vi "DAQ_Vibration (SubVI).vi"(8 "error in (no error)":errorcluster, 11 "output cluster":T1) -> (0 "error out":errorcluster)   [LabVIEW 2016]
uses:
  Que Cluster TD.ctl
  Que Attributes TD.ctl
  Que enum td.ctl
  Vibration data TD.ctl
  <vilib>/DAQmx/read.llb/DAQmx Read (Analog 2D DBL NChan NSamp).vi
  <vilib>/DAQmx/miscellaneous.llb/DAQmx Fill In Error Info.vi
  <resource>/objmgr/daqmx.rc
panel:
  out "Vibration_2":dbl[][](graph)
  out "Vibration_1":dbl[][](graph)
  in  "samples per read operation":i32=2560
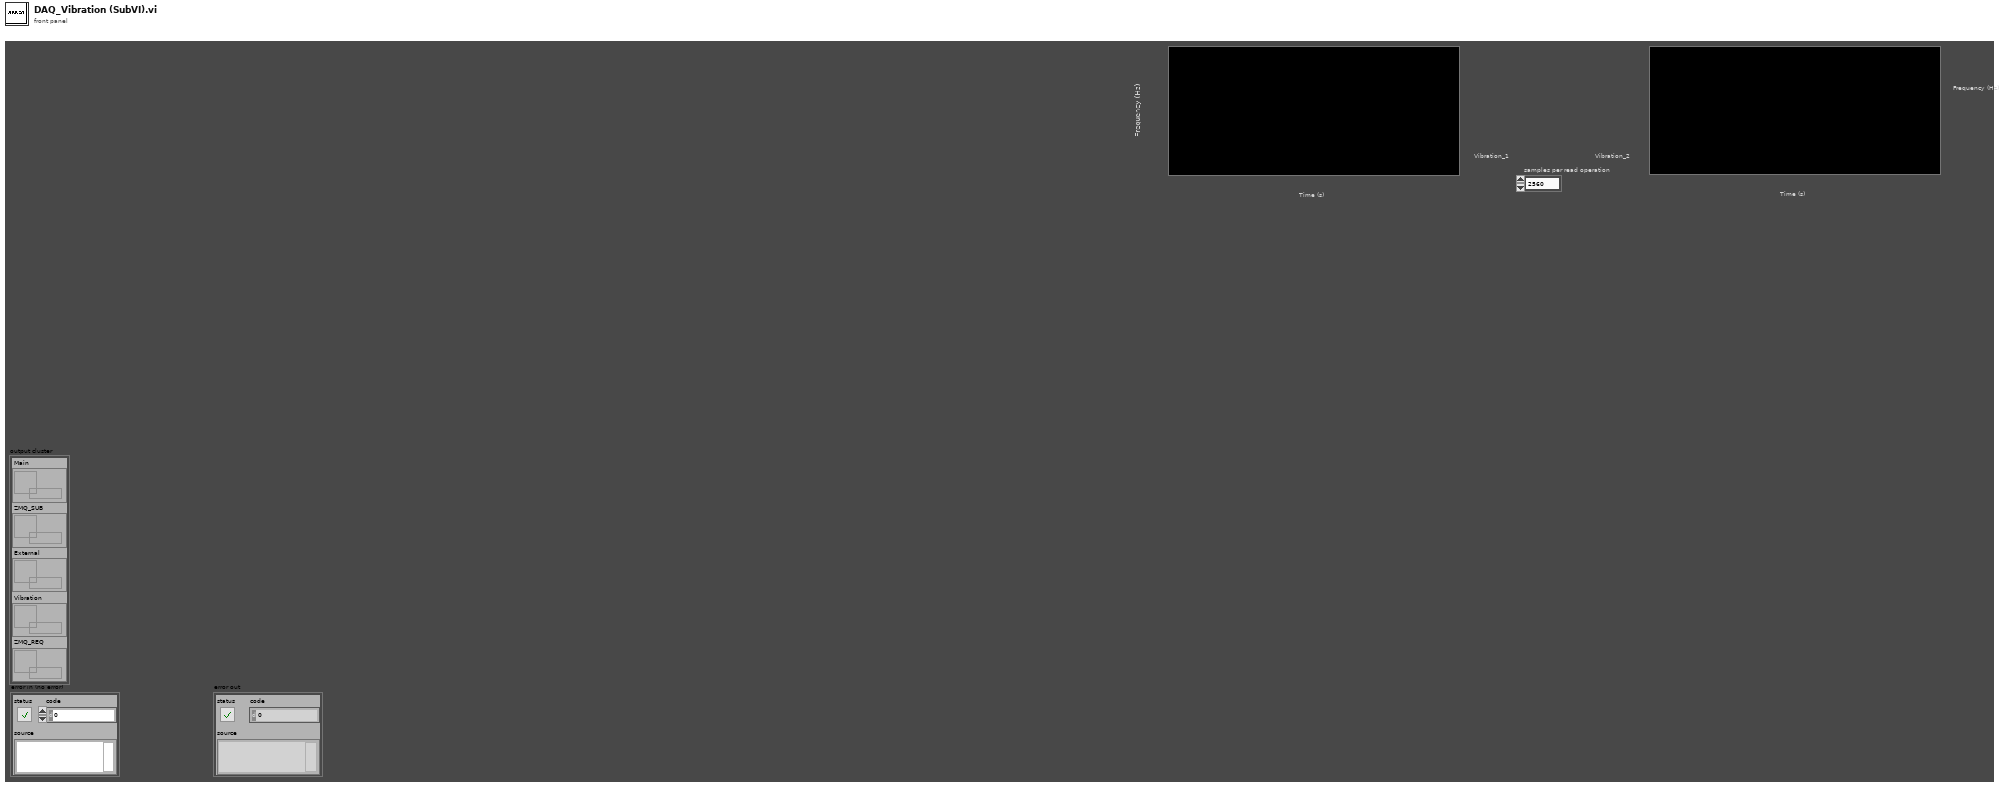
[diagram p1: front panel]
types:
  T1 = typedef "Que Cluster TD.ctl" = cluster{"Main":refnum<queue>, "ZMQ_SUB":refnum<queue>, "External":refnum<queue>, "Vibration":refnum<queue>, "ZMQ_REQ":refnum<queue>}
  T2 = typedef "Vibration data TD.ctl" = cluster{"# samples":i32, "Vibration_1":dbl[], "Vibration_2":dbl[], "Connected?":bool, "Logging?":bool, "TimeStamp":dbl, "Data":dbl[][], "LogFilePath":path}
  T3 = typedef "Que Attributes TD.ctl" = cluster{"Que States":T4, "String":string, "Boolean":bool, "Double":dbl, "U16":u16}
  T4 = typedef "Que enum td.ctl" = enum16{"Stop", "Start", "Update D_HW", "Initialize", "Exit", "Read", "Write", "Plot", "Log", "Stop Log", "Start Log", "Wait"}
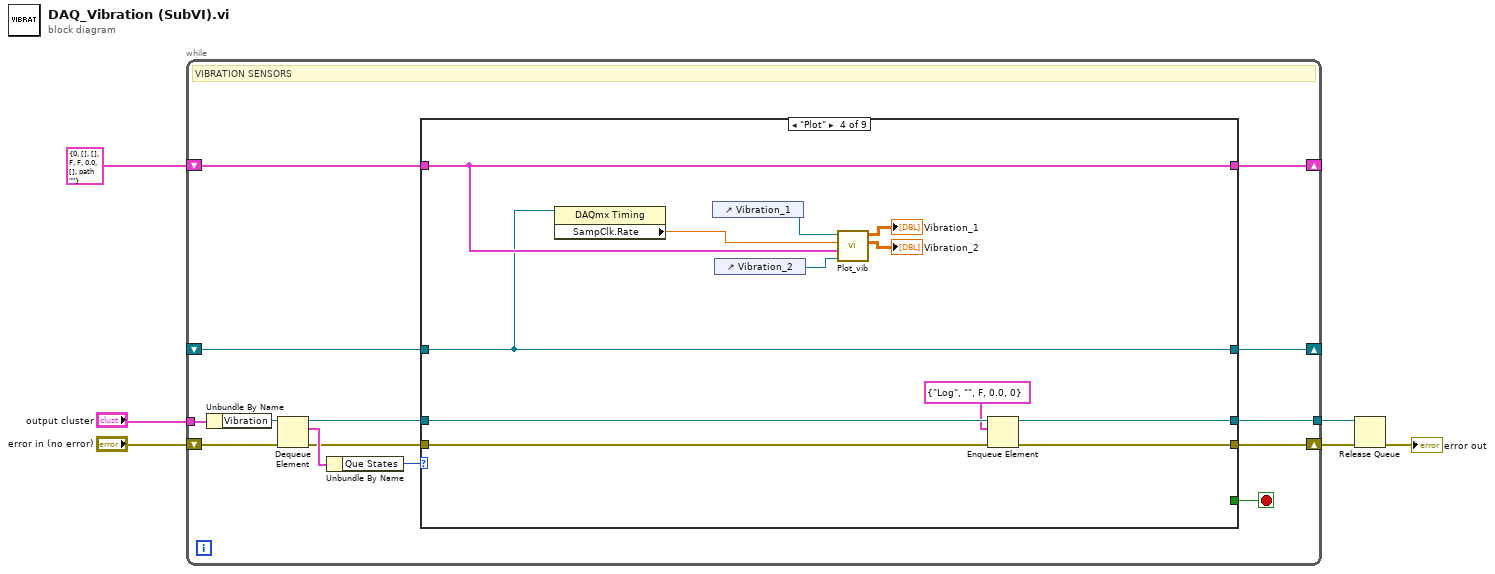
[diagram p0: block diagram]
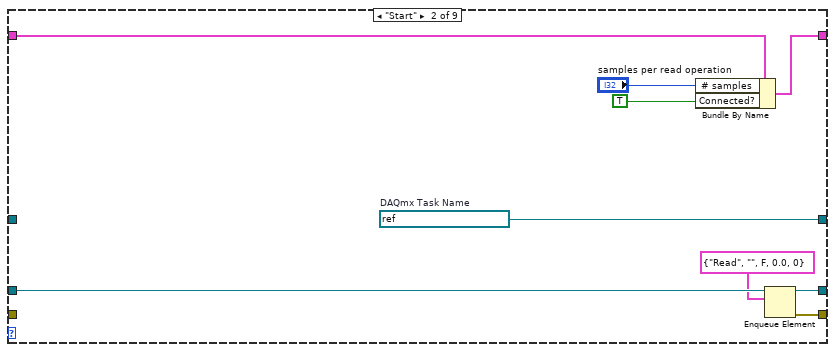
[diagram p3: hidden frame]
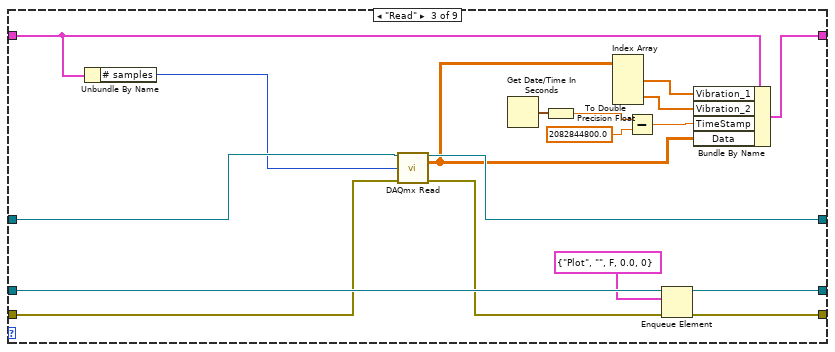
[diagram p4: hidden frame]
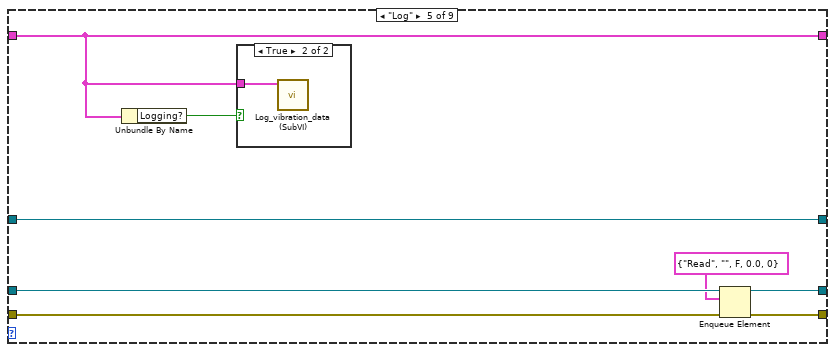
[diagram p5: hidden frame]
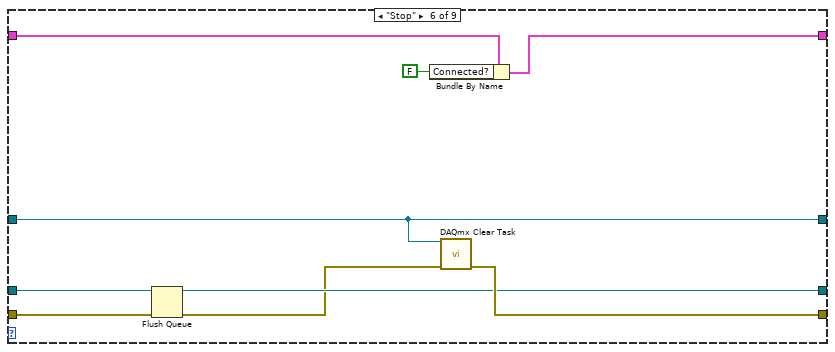
[diagram p7: hidden frame]
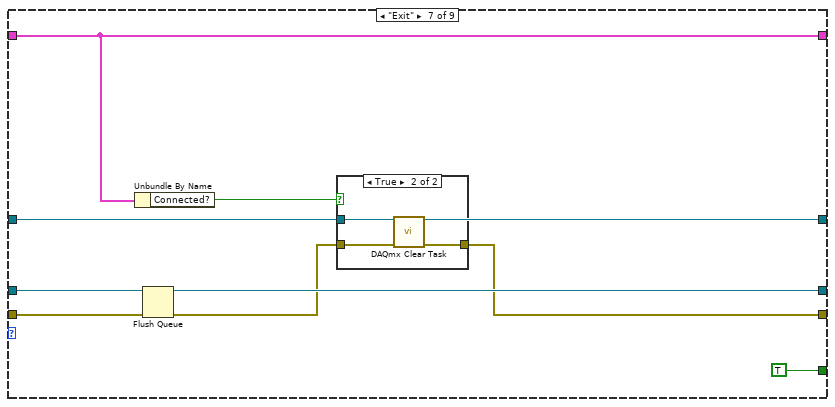
[diagram p8: hidden frame]
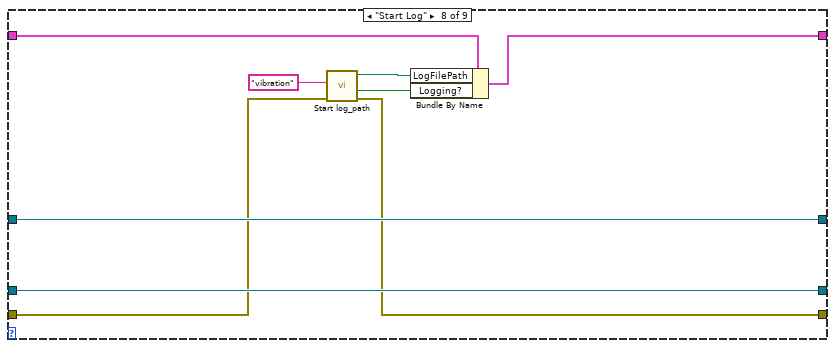
[diagram p10: hidden frame]
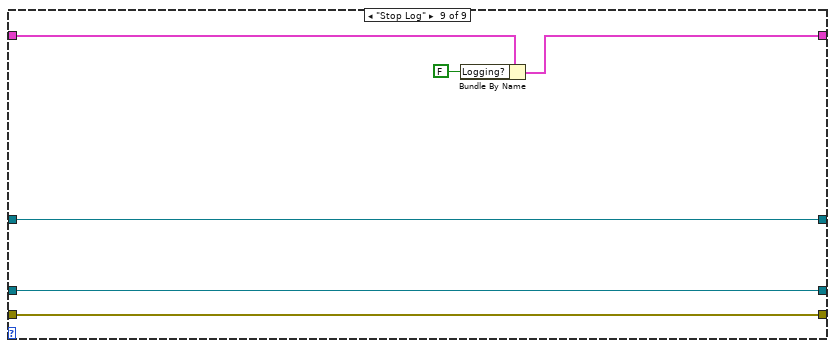
[diagram p11: hidden frame]
diagram:
  n1 = while {
    tunnel: "output cluster" -> [w20]
    tunnel: [w14] -> w5
    shift-right: [w13] -> w6
    shift-left: "error in (no error)" -> [w18]
    shift-right: [w10] -> _
    shift-left: _ -> [w9]
    shift-right: [w7] -> _
    shift-left: T2 {"# samples"=0, "Vibration_1"=[], "Vibration_2"=[], "Connected?"=FALSE, "Logging?"=FALSE, "TimeStamp"=0.0, "Data"=[], "LogFilePath"=path ""} ("External Data TD") -> [w8]
    stop <- w11 stop-if-true
    # "VIBRATION SENSORS"
    n2 = Unbundle By Name(w20) -> ("Vibration"=w19:refnum<queue>)
    n3 = Dequeue Element(queue=w19, error in (no error)=w18) -> (queue out=w15:refnum<queue>, element=w17:T3, error out=w16:errorcluster)  [unwired: 1 in, 1 out]
    n4 = Unbundle By Name(w17) -> ("Que States"=w12:T4)
    n5 = case shown="\"Plot\"" w12 {
      tunnel: w16 -> [w21 _ w47 w61 w67 w77 w84 w98 w104]
      tunnel: w15 -> [w22 w32 w50 w63 w69 w76 w86 w103 w109]
      tunnel: [w22 w31 w49 w62 w68 w75 w85 w103 w109] -> w14
      tunnel: [w21 w33 w51 w60 w66 w78 w82 w97 w104] -> w13
      tunnel: [_ _ _ _ _ _ TRUE _ _] -> w11
      tunnel: [w24 w25 w45 w53 w71 w73 w89 w102 w108] -> w10
      tunnel: w9 -> [w24 _ w39 w53 w71 w73 w89 w102 w108]
      tunnel: w8 -> [w23 w29 w38 w56 w64 w81 w88 w101 w107]
      tunnel: [w23 w28 w44 w56 w64 w80 w88 w100 w106] -> w7
      frame "Initialize", Default {
      }
      frame "Start" {
        w25 = refnum<k21> "Accelerometers_Task"  # DAQmx Task Name
        n6 = Bundle By Name(cluster=w29, "# samples"="samples per read operation", "Connected?"=TRUE) -> (w28:T2)
        n7 = Enqueue Element(queue=w32, element=T3 {"Que States"=enum."Read", "String"="", "Boolean"=FALSE, "Double"=0.0, "U16"=0}) -> (queue out=w31:refnum<queue>, error out=w33:errorcluster)  [unwired: 2 in, 1 out]
      }
      frame "Read" {
        n8 = Unbundle By Name(w38) -> ("# samples"=w37:i32)
        n9 = call-poly <vilib>:"DAQmx Read.vi"("task/channels in"=w39, "number of samples per channel"=w37, "error in"=w47) -> ("task out"=w45:refnum<k21>, "data"=w36:dbl[][], "error out"=w46:errorcluster)  [unwired: 10 in]
        n10 = Get Date/Time In Seconds() -> (seconds since 1Jan1904=w43:timestamp)
        n11 = To Double Precision Float(number=w43) -> (double precision float=w42:dbl)
        n12 = Index Array(array=w36) -> (element #1=w35:dbl[], element #2=w34:dbl[])  [unwired: 4 in]
        n13 = Subtract(x=w42, y=2082844800.0 ("Epoch Delta (s)")) -> (x-y=w40:dbl)
        n14 = Enqueue Element(queue=w50, element=T3 {"Que States"=enum."Plot", "String"="", "Boolean"=FALSE, "Double"=0.0, "U16"=0}, error in (no error)=w46) -> (queue out=w49:refnum<queue>, error out=w51:errorcluster)  [unwired: 1 in, 1 out]
        n15 = Bundle By Name(cluster=w38, "Vibration_1"=w35, "Vibration_2"=w34, "TimeStamp"=w40, "Data"=w36) -> (w44:T2)
      }
      frame "Plot" {
        n16 = property class="DAQmx Timing"(reference=w53) -> ("SampClk.Rate"=w52:dbl)  [unwired: 1 in, 2 out]
        n17 = control-ref of="Vibration_1"() -> (w57:refnum<vi>)
        n18 = control-ref of="Vibration_2"() -> (w54:refnum<vi>)
        n19 = call "Plot_vib.vi"("IntensityGraph in 2"=w54, "External Data TD"=w56, "sampling rate"=w52, "IntensityGraph in"=w57) -> ("STFT Spectrogram 2"=→"Vibration_2":dbl[][], "STFT Spectrogram"=→"Vibration_1":dbl[][])  [unwired: 6 in]
        n20 = Enqueue Element(queue=w63, element=T3 {"Que States"=enum."Log", "String"="", "Boolean"=FALSE, "Double"=0.0, "U16"=0}, error in (no error)=w61) -> (queue out=w62:refnum<queue>, error out=w60:errorcluster)  [unwired: 1 in, 1 out]
      }
      frame "Log" {
        n21 = Unbundle By Name(w64) -> ("Logging?"=w70:bool)
        n22 = case shown="True" w70 {
          tunnel: w64 -> [_ w72]
          frame False {
          }
          frame True {
            n23 = call "Log_vibration_data (SubVI).vi"("vibration Data TD"=w72) -> ()  [unwired: 11 in]
          }
        }
        n24 = Enqueue Element(queue=w69, element=T3 {"Que States"=enum."Read", "String"="", "Boolean"=FALSE, "Double"=0.0, "U16"=0}, error in (no error)=w67) -> (queue out=w68:refnum<queue>, error out=w66:errorcluster)  [unwired: 1 in, 1 out]
      }
      frame "Stop" {
        n25 = Flush Queue(queue=w76, error in (no error)=w77) -> (queue out=w75:refnum<queue>, error out=w74:errorcluster)  [unwired: 1 out]
        n26 = Bundle By Name(cluster=w81, "Connected?"=FALSE) -> (w80:T2)
        n27 = call <vilib>:"DAQmx Clear Task.vi"("task in"=w73, "error in"=w74) -> ("error out"=w78:errorcluster)  [unwired: 13 in]
      }
      frame "Exit" {
        n28 = Unbundle By Name(w88) -> ("Connected?"=w87:bool)
        n29 = Flush Queue(queue=w86, error in (no error)=w84) -> (queue out=w85:refnum<queue>, error out=w83:errorcluster)  [unwired: 1 out]
        n30 = case shown="True" w87 {
          tunnel: w89 -> [_ w94]
          tunnel: w83 -> [w91 w93]
          tunnel: [w91 w92] -> w82
          frame False {
          }
          frame True {
            n31 = call <vilib>:"DAQmx Clear Task.vi"("task in"=w94, "error in"=w93) -> ("error out"=w92:errorcluster)  [unwired: 13 in]
          }
        }
      }
      frame "Start Log" {
        n32 = call "Start log_path.vi"("error in (no error)"=w98, "Filename root"="vibration" ("Data type")) -> ("error out"=w97:errorcluster, "Logging"=w99:bool, "Path"=w95:path)  [unwired: 7 in]
        n33 = Bundle By Name(cluster=w101, "LogFilePath"=w95, "Logging?"=w99) -> (w100:T2)
      }
      frame "Stop Log" {
        n34 = Bundle By Name(cluster=w107, "Logging?"=FALSE) -> (w106:T2)
      }
    }
  }
  n35 = Release Queue(queue=w5, error in (no error)=w6) -> (error out=→"error out":errorcluster)  [unwired: 1 in, 2 out]
